vi "Termometr0-2 (SubVI).vi"(11 "Numeric":dbl) -> (3 "Град":dbl)   [LabVIEW 2020]
uses:
  <vilib>/numeric/Random Number (Range) I64.vi
  <vilib>/numeric/sub_Random U32.vi
panel:
  out "Numeric 2":dbl
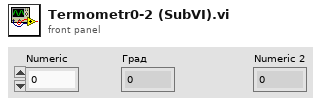
[diagram p1: front panel]
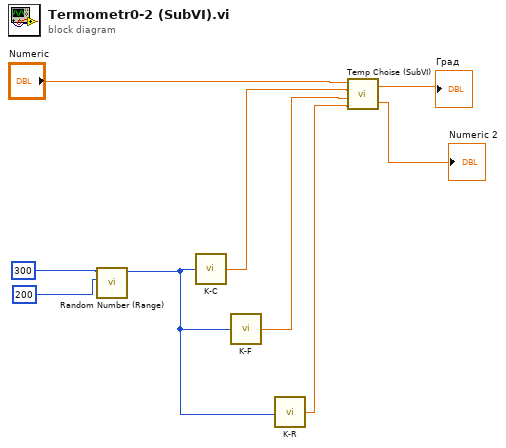
[diagram p0: block diagram]
diagram:
  n1 = call-poly <vilib>:"Random Number (Range).vi"("lower bound (-100)"=200, "upper bound (100)"=300) -> ("number"=w9:i64)  [unwired: 9 in]
  n2 = call "K-C.vi"("Град F"=w9) -> ("Град C"=w5:dbl)
  n3 = call "K-F.vi"("Град K"=w9) -> ("Град F"=w4:dbl)
  n4 = call "K-R.vi"("Град K"=w9) -> ("Град R"=w3:dbl)
  n5 = call "Temp Choise (SubVI).vi"("R"=w3, "F"=w4, "C"=w5, "Numeric"="Numeric") -> ("Numeric 2"=→"Numeric 2":dbl, "temp"=→"Град":dbl)
